vi "Save_Universal.vi"(9 "Directory Path":path=path "I:/Temporary", 11 "Data to be Save":variant[](array[variant])=[variant(string "")]) -> ()   [LabVIEW 2020]
uses:
  <vilib>/Utility/Data Type/Type Definitions/Data Type.ctl
  <vilib>/Utility/file.llb/Write Delimited Spreadsheet (DBL).vi
  <vilib>/Utility/file.llb/Write Delimited Spreadsheet (I64).vi
  <vilib>/Utility/Data Type/NI_Data Type.lvlib
panel:
  out "Array 2":T1[](array[typedef])
  out "name":string="Stringde"
  out "error out":errorcluster={"status"=TRUE, "code"=7, "source"="Open/Create/Replace File in Save_Universal.vi<APPEND>\n2021_09_06 17_44_50.md:\\"}
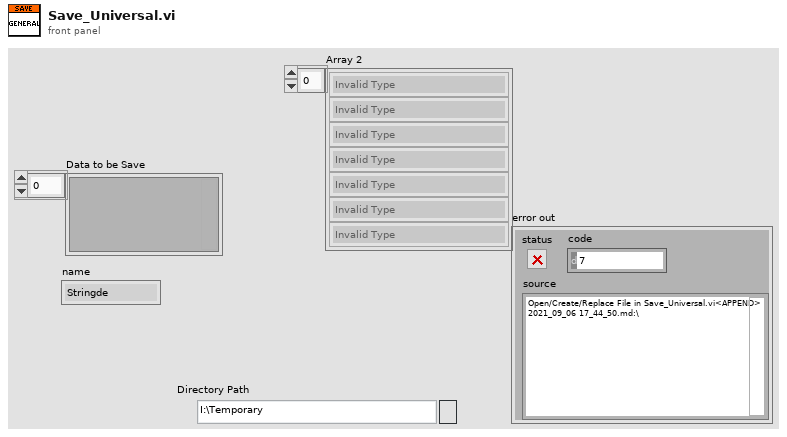
[diagram p1: front panel]
types:
  T1 = typedef "NI_Data Type.lvlib/Data Type.ctl" = enum8{"Invalid Type", "Void", "I8", "I16", "I32", "I64", "U8", "U16", "U32", "U64", "Single Float", "Double Float", "Extended Float", "Single Complex", "Double Complex", "Extended Complex", "Enum U8", "Enum U16", "Enum U32", "Enum U64", "Single Float With Unit", "Double Float With Unit", "Extended Float With Unit", "Single Complex with Unit", "Double Complex with Unit", "Extended Complex with Unit", "Boolean", "String", "Path", "Picture", "Tag", "Array", "Cluster", "Variant", "LV Variant", "Waveform", "Timestamp", "Digital Waveform", "Digital Data", "ExpressData", "Refnum", "External Data", "VI", "Poly VI", "LabVIEW Class Instance", "Fixed Point", "Set Collection", "Map Collection"}
  T2 = enum16{"open", "replace", "create", "open or create", "replace or create", "replace or create with confirmation"}
  T3 = typedef "NI_Data Type.lvlib/Refnum Type.ctl" = enum16{"NotARefnum", "UnknownRefnum", "Generic", "Datalog", "ByteStream", "Device", "Occurence", "TCPNetConnection", "Auto", "Menu", "Imaq", "Hardware", "DataSocket", "Visa", "IVI", "UDPNetConnection", "Notifier", "Queue", "Irda", "EventReg", "DotNet", "UserEvent", "Callback", "UNUSED_EMPTY_POSITION", "BlueToothNetConnection", "LVObjApp", "LVObjVI", "LVObjUnknown", "GenericClass", "UserDefinedRefnumTag", "DataValue", "RT FIFO", "TDMS File", "PythonSessionRefnum"}
  T4 = typedef "imagedata.ctl" = cluster{"image type":i32, "image depth":i32, "image":u8[], "mask":u8[], "colors":u32[], "Rectangle":cluster{"left":i16, "top":i16, "right":i16, "bottom":i16}}
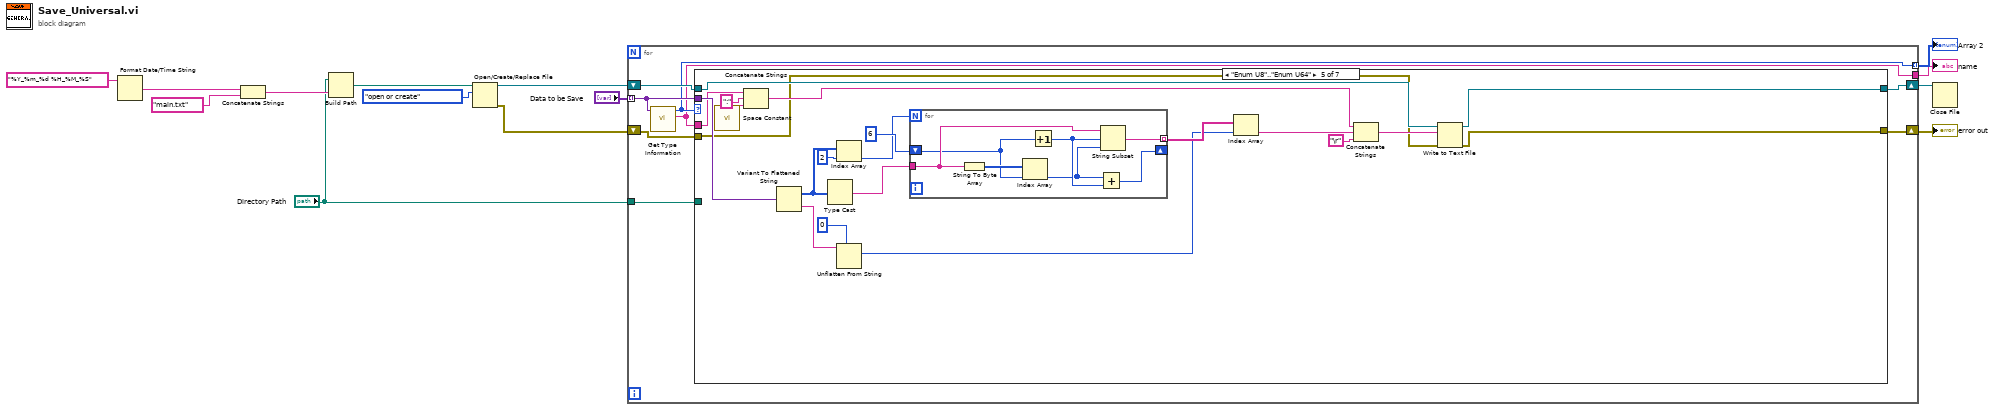
[diagram p0: block diagram]
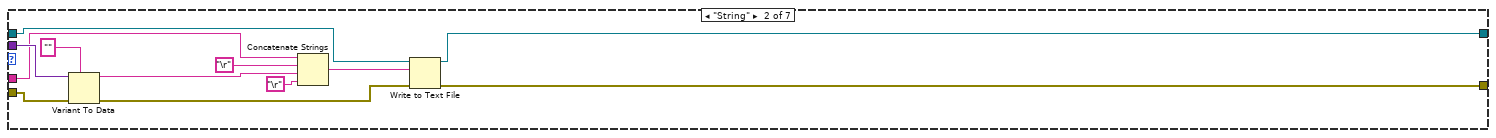
[diagram p3: hidden frame]
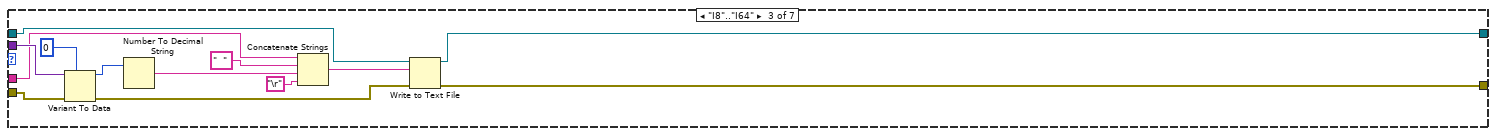
[diagram p4: hidden frame]
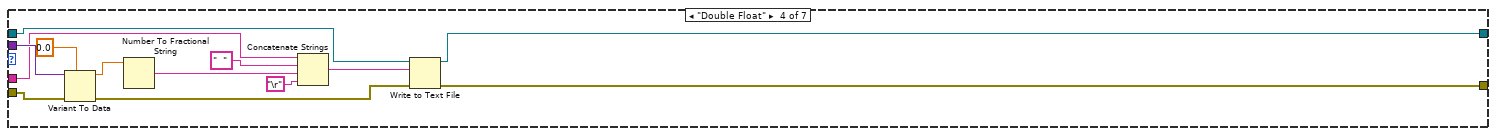
[diagram p5: hidden frame]
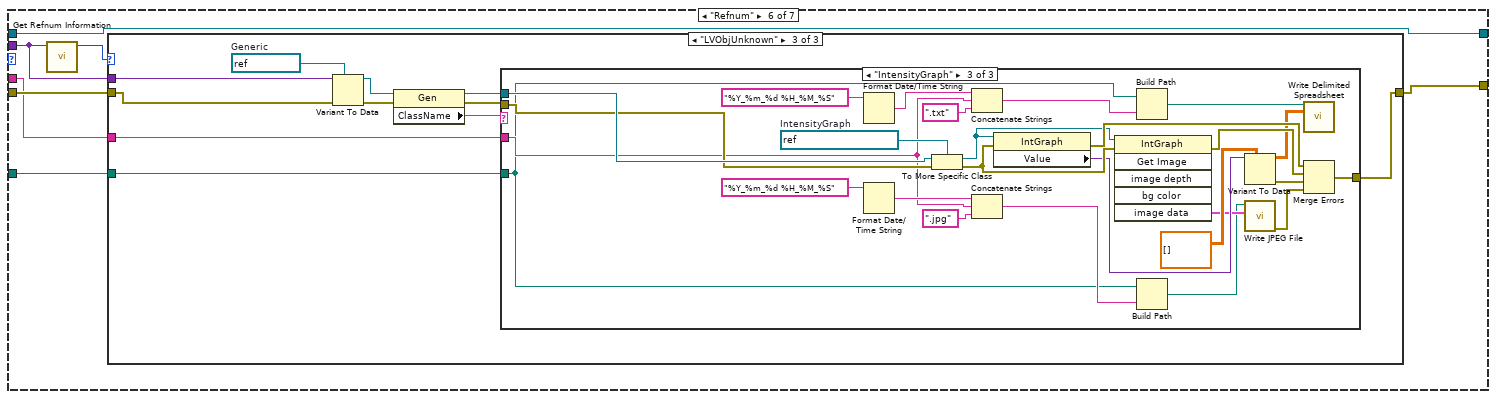
[diagram p6: hidden frame]
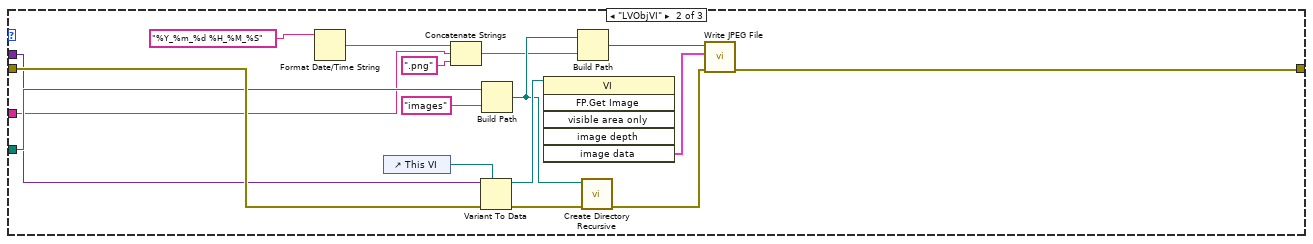
[diagram p8: hidden frame]
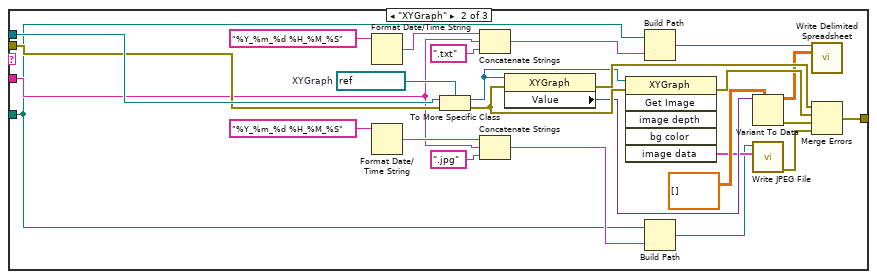
[diagram p10: hidden frame]
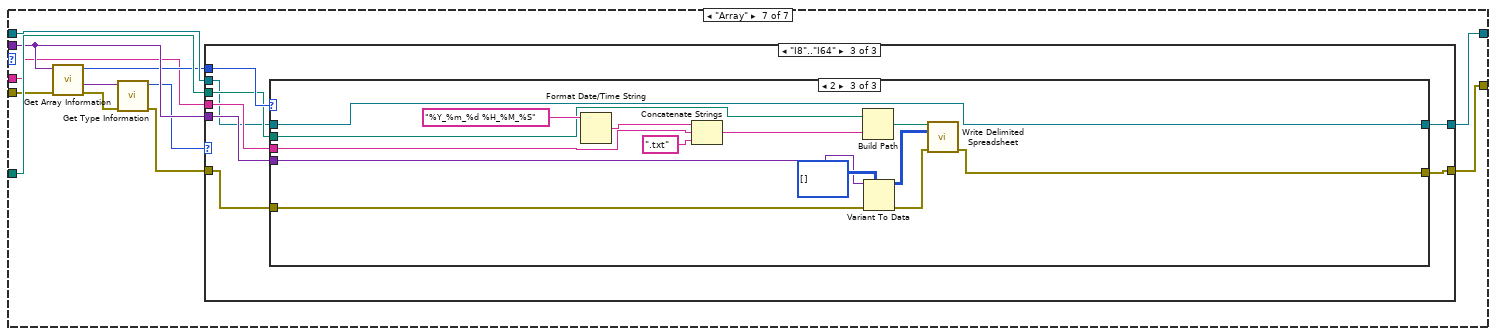
[diagram p11: hidden frame]
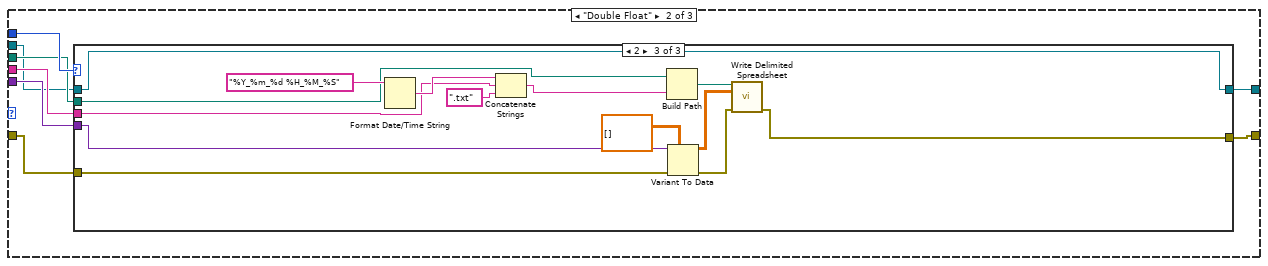
[diagram p13: hidden frame]
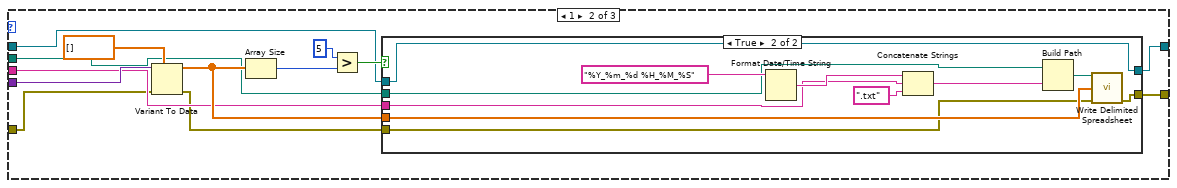
[diagram p15: hidden frame]
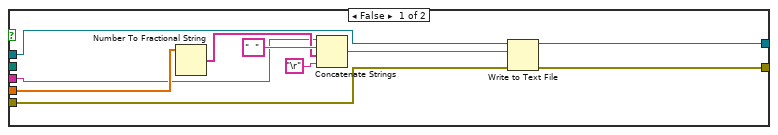
[diagram p16: hidden frame]
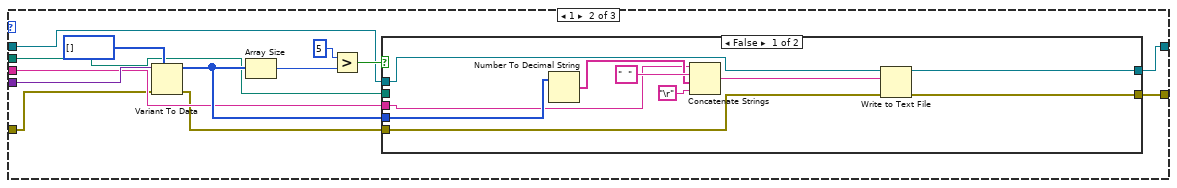
[diagram p18: hidden frame]
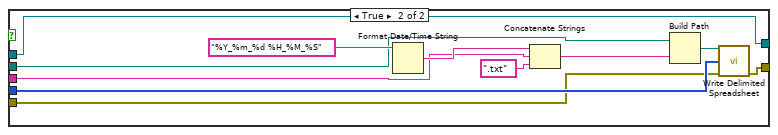
[diagram p19: hidden frame]
diagram:
  n1 = Format Date/Time String(time format string (%c)="%Y_%m_%d %H_%M_%S") -> (date/time string=w11:string)  [unwired: 2 in]
  n2 = Concatenate Strings(w11, "main.txt" ("string")) -> (w9:string)
  n3 = Build Path(base path="Directory Path", name or relative path=w9) -> (appended path=w10:path)
  n4 = Open/Create/Replace File(file path (use dialog)=w10, operation (0:open)=T2."open or create") -> (refnum out=w8:refnum<file>, error out=w7:errorcluster)  [unwired: 4 in, 1 out]
  n5 = for {
    tunnel: "Data to be Save" -> [w21] mode=indexing
    shift-right: [w19] -> w4
    shift-left: w8 -> [w22]
    shift-right: [w18] -> w6
    shift-left: w7 -> [w20]
    tunnel: "Directory Path" -> [w17]
    tunnel: [w16] -> w2 mode=indexing
    tunnel: [w15] -> w1
    n6 = call <vilib>:"Get Type Information.vi"("variant"=w21) -> ("name"=w15:string, "type"=w16:T1)  [unwired: 6 in, 3 out]
    n7 = case shown="\"Enum U8\"..\"Enum U64\"" w16 {
      tunnel: w15 -> [_ w33 w39 w54 w65 w91 w181]
      tunnel: w22 -> [w24 w30 w43 w58 w83 w94 w184]
      tunnel: w21 -> [_ w35 w47 w60 w68 w92 w188]
      tunnel: w20 -> [w23 w34 w42 w57 w63 w97 w180]
      tunnel: [w24 w28 w40 w55 w82 w94 w183] -> w19
      tunnel: [w23 w26 w41 w56 w80 w95 w189] -> w18
      tunnel: w17 -> [_ _ _ _ _ w96 w190]
      frame "Invalid Type", Default {
      }
      frame "String" {
        n8 = Variant To Data(error in=w34, type="", Variant=w35) -> (data=w32:string, error out=w27:errorcluster)
        n9 = Concatenate Strings(w33, "\r", w32, "\r") -> (w29:string)
        n10 = Write to Text File(file (use dialog)=w30, text=w29, error in=w27) -> (refnum out=w28:refnum<file>, error out=w26:errorcluster)  [unwired: 1 in, 1 out]
      }
      frame "I8".."I64" {
        n11 = Variant To Data(error in=w42, type=0, Variant=w47) -> (data=w44:i32, error out=w49:errorcluster)
        n12 = Number To Decimal String(number=w44) -> (decimal integer string=w45:string)  [unwired: 1 in]
        n13 = Concatenate Strings(w39, "  " ("string"), w45, "\r") -> (w48:string)
        n14 = Write to Text File(file (use dialog)=w43, text=w48, error in=w49) -> (refnum out=w40:refnum<file>, error out=w41:errorcluster)  [unwired: 1 in, 1 out]
      }
      frame "Double Float" {
        n15 = Variant To Data(error in=w57, type=0.0, Variant=w60) -> (data=w52:dbl, error out=w62:errorcluster)
        n16 = Number To Fractional String(number=w52) -> (F-format string=w51:string)  [unwired: 3 in]
        n17 = Concatenate Strings(w54, "  " ("string"), w51, "\r") -> (w61:string)
        n18 = Write to Text File(file (use dialog)=w58, text=w61, error in=w62) -> (refnum out=w55:refnum<file>, error out=w56:errorcluster)  [unwired: 1 in, 1 out]
      }
      frame "Enum U8".."Enum U64" {
        n19 = call <vilib>:"Space Constant.vi"() -> ("String"=w81:string)
        n20 = Concatenate Strings(w65, ":" ("string"), w81) -> (w66:string)
        n21 = Variant To Flattened String(Variant=w68) -> (data string=w77:string, 1:w71:i16[])
        n22 = Type Cast(x=w71) -> (*(type *) &x=w75:string)  [unwired: 1 in]
        n23 = Index Array(array=w71, index=2) -> (element=w69:i16)
        n24 = Unflatten From String(type=u16 0, binary string=w77) -> (value=w72:u16)  [unwired: 3 in, 2 out]
        n25 = for {
          N: w69 -> [_]
          tunnel: w75 -> [w87]
          shift-right: [w86] -> _
          shift-left: 6 ("index") -> [w84]
          tunnel: [w85] -> w73 mode=indexing
          n26 = String To Byte Array(string=w87) -> (unsigned byte array=w90:u8[])
          n27 = Index Array(array=w90, index=w84) -> (element=w88:u8)
          n28 = Increment(x=w84) -> (x+1=w89:i32)
          n29 = Add(x=w88, y=w89) -> (x+y=w86:i32)
          n30 = String Subset(string=w87, offset (0)=w89, length (rest)=w88) -> (substring=w85:string)
        }
        n31 = Index Array(array=w73, index=w72) -> (element=w67:string)
        n32 = Concatenate Strings(w66, w67, "\r") -> (w79:string)
        n33 = Write to Text File(file (use dialog)=w83, text=w79, error in=w63) -> (refnum out=w82:refnum<file>, error out=w80:errorcluster)  [unwired: 1 in, 1 out]
      }
      frame "Refnum" {
        n34 = call <vilib>:"Get Refnum Information.vi"("variant"=w92) -> ("reference type"=w93:T3)  [unwired: 7 in, 3 out]
        n35 = case shown="\"LVObjUnknown\"" w93 {
          tunnel: w97 -> [w98 w113 w123]
          tunnel: w96 -> [_ w109 w116]
          tunnel: [w98 w108 w118] -> w95
          tunnel: w92 -> [_ w107 w125]
          tunnel: w91 -> [_ w99 w117]
          frame "NotARefnum", Default {
          }
          frame "LVObjVI" {
            n36 = Format Date/Time String(time format string (%c)="%Y_%m_%d %H_%M_%S") -> (date/time string=w100:string)  [unwired: 2 in]
            n37 = control-ref of="This VI"() -> (w115:refnum<vi>)
            n38 = Concatenate Strings(w100, w99, ".png" ("string")) -> (w102:string)
            n39 = Variant To Data(error in=w113, type=w115, Variant=w107) -> (data=w112:refnum<vi>, error out=w106:errorcluster)
            n40 = Build Path(base path=w109, name or relative path="images" ("string")) -> (appended path=w104:path)
            n41 = invoke class="VI" method="FP.Get Image"(reference=w112) -> ("image data"=w114:T4)  [unwired: 5 in, 5 out]
            n42 = Build Path(base path=w104, name or relative path=w102) -> (appended path=w101:path)
            n43 = call <vilib>:"Create Directory Recursive.vi"("error in (no error)"=w106, "directory"=w104) -> ("error out"=w105:errorcluster)  [unwired: 3 in, 2 out]
            n44 = call <vilib>:"Write JPEG File.vi"("error in (no error)"=w105, "image data"=w114, "path to JPEG file"=w101) -> ("error out"=w108:errorcluster)  [unwired: 8 out]
          }
          frame "LVObjUnknown" {
            w126 = refnum<vi> refnum  # Generic
            n45 = Variant To Data(error in=w123, type=w126, Variant=w125) -> (data=w124:refnum<vi>, error out=w122:errorcluster)
            n46 = property class="Gen"(reference=w124, error in=w122) -> (reference out=w120:refnum<vi>, error out=w119:errorcluster, "ClassName"=w121:string)
            n47 = case shown="\"IntensityGraph\"" w121 {
              tunnel: w120 -> [_ w151 w177]
              tunnel: w119 -> [_ w150 w176]
              tunnel: [_ w146 w172] -> w118
              tunnel: w117 -> [_ w133 w159]
              tunnel: w116 -> [_ w130 w156]
              frame "False", Default {
              }
              frame "XYGraph" {
                w152 = refnum<vi> refnum  # XYGraph
                n48 = Format Date/Time String(time format string (%c)="%Y_%m_%d %H_%M_%S") -> (date/time string=w138:string)  [unwired: 2 in]
                n49 = Format Date/Time String(time format string (%c)="%Y_%m_%d %H_%M_%S") -> (date/time string=w135:string)  [unwired: 2 in]
                n50 = To More Specific Class(target class=w152, reference=w151, error in=w150) -> (specific class reference=w145:refnum<vi>, error out=w149:errorcluster)
                n51 = Concatenate Strings(w138, w133, ".txt" ("string")) -> (w136:string)
                n52 = Concatenate Strings(w135, w133, ".jpg" ("string")) -> (w131:string)
                n53 = property class="XYGraph"(reference=w145, error in=w149) -> (error out=w148:errorcluster, "Value"=w144:variant)  [unwired: 1 out]
                n54 = invoke class="XYGraph" method="Get Image"(reference=w145, error in=w149) -> (error out=w147:errorcluster, "image data"=w132:T4)  [unwired: 4 in, 4 out]
                n55 = Build Path(base path=w130, name or relative path=w136) -> (appended path=w137:path)
                n56 = Build Path(base path=w130, name or relative path=w131) -> (appended path=w129:path)
                n57 = Variant To Data(type=dbl[][] [] ("1D data"), Variant=w144) -> (data=w142:dbl[][], error out=w143:errorcluster)  [unwired: 1 in]
                n58 = call <vilib>:"Write JPEG File.vi"("image data"=w132, "path to JPEG file"=w129) -> ("error out"=w128:errorcluster)  [unwired: 1 in, 8 out]
                n59 = call-poly <vilib>:"Write Delimited Spreadsheet.vi"("file path (dialog if empty)"=w137, "2D data"=w142) -> ()  [unwired: 12 in, 2 out]
                n60 = Merge Errors(w148, w147, w143, w128) -> (w146:errorcluster)
              }
              frame "IntensityGraph" {
                w178 = refnum<vi> refnum  # IntensityGraph
                n61 = Format Date/Time String(time format string (%c)="%Y_%m_%d %H_%M_%S") -> (date/time string=w164:string)  [unwired: 2 in]
                n62 = Format Date/Time String(time format string (%c)="%Y_%m_%d %H_%M_%S") -> (date/time string=w161:string)  [unwired: 2 in]
                n63 = To More Specific Class(target class=w178, reference=w177, error in=w176) -> (specific class reference=w171:refnum<vi>, error out=w175:errorcluster)
                n64 = Concatenate Strings(w164, w159, ".txt" ("string")) -> (w162:string)
                n65 = Concatenate Strings(w161, w159, ".jpg" ("string")) -> (w157:string)
                n66 = property class="IntGraph"(reference=w171, error in=w175) -> (error out=w174:errorcluster, "Value"=w170:variant)  [unwired: 1 out]
                n67 = invoke class="IntGraph" method="Get Image"(reference=w171, error in=w175) -> (error out=w173:errorcluster, "image data"=w158:T4)  [unwired: 4 in, 4 out]
                n68 = Build Path(base path=w156, name or relative path=w162) -> (appended path=w163:path)
                n69 = Build Path(base path=w156, name or relative path=w157) -> (appended path=w155:path)
                n70 = Variant To Data(type=dbl[][] [] ("1D data"), Variant=w170) -> (data=w168:dbl[][], error out=w169:errorcluster)  [unwired: 1 in]
                n71 = call <vilib>:"Write JPEG File.vi"("image data"=w158, "path to JPEG file"=w155) -> ("error out"=w154:errorcluster)  [unwired: 1 in, 8 out]
                n72 = call-poly <vilib>:"Write Delimited Spreadsheet.vi"("file path (dialog if empty)"=w163, "2D data"=w168) -> ()  [unwired: 12 in, 2 out]
                n73 = Merge Errors(w174, w173, w169, w154) -> (w172:errorcluster)
              }
            }
          }
        }
      }
      frame "Array" {
        n74 = call <vilib>:"Get Array Information.vi"("error in (no error)"=w180, "variant"=w188) -> ("error out"=w187:errorcluster, "array element data type"=w186:variant, "number of dimensions"=w182:i32)  [unwired: 6 in, 1 out]
        n75 = call <vilib>:"Get Type Information.vi"("error in (no error)"=w187, "variant"=w186) -> ("error out"=w179:errorcluster, "type"=w185:T1)  [unwired: 5 in, 3 out]
        n76 = case shown="\"I8\"..\"I64\"" w185 {
          tunnel: w179 -> [w192 w196 w254]
          tunnel: w190 -> [_ w198 w256]
          tunnel: [w192 w195 w253] -> w189
          tunnel: w188 -> [_ w197 w255]
          tunnel: w184 -> [w191 w193 w251]
          tunnel: [w191 w194 w252] -> w183
          tunnel: w182 -> [_ w200 w258]
          tunnel: w181 -> [_ w199 w257]
          frame "Invalid Type", Default {
          }
          frame "Double Float" {
            n77 = case shown="2" w200 {
              tunnel: w199 -> [_ w208 w248]
              tunnel: w198 -> [_ w209 w245]
              tunnel: w197 -> [_ w214 w242]
              tunnel: w196 -> [w201 w206 w241]
              tunnel: [w201 w204 w238] -> w195
              tunnel: w193 -> [w202 w207 w237]
              tunnel: [w202 w203 w237] -> w194
              frame 0, Default {
              }
              frame 1 {
                n78 = Variant To Data(error in=w206, type=dbl[] [] ("1D data"), Variant=w214) -> (data=w210:dbl[], error out=w205:errorcluster)
                n79 = Array Size(array=w210) -> (size(s)=w213:i32)
                n80 = Greater?(x=5, y=w213) -> (0:w211:bool)
                n81 = case shown="True" w211 {
                  tunnel: w210 -> [w221 w236]
                  tunnel: w209 -> [_ w231]
                  tunnel: w208 -> [w218 w229]
                  tunnel: w207 -> [w217 w228]
                  tunnel: w205 -> [w220 w227]
                  tunnel: [w219 w226] -> w204
                  tunnel: [w216 w228] -> w203
                  frame False {
                    n82 = Number To Fractional String(number=w221) -> (F-format string=w223:string[])  [unwired: 3 in]
                    n83 = Concatenate Strings(w218, "  " ("string"), w223, "\r") -> (w225:string)
                    n84 = Write to Text File(file (use dialog)=w217, text=w225, error in=w220) -> (refnum out=w216:refnum<file>, error out=w219:errorcluster)  [unwired: 1 in, 1 out]
                  }
                  frame True {
                    n85 = Format Date/Time String(time format string (%c)="%Y_%m_%d %H_%M_%S") -> (date/time string=w235:string)  [unwired: 2 in]
                    n86 = Concatenate Strings(w235, w229, ".txt" ("string")) -> (w232:string)
                    n87 = Build Path(base path=w231, name or relative path=w232) -> (appended path=w230:path)
                    n88 = call-poly <vilib>:"Write Delimited Spreadsheet.vi"("file path (dialog if empty)"=w230, "1D data"=w236, "error in (no error)"=w227) -> ("error out"=w226:errorcluster)  [unwired: 11 in, 1 out]
                  }
                }
              }
              frame 2 {
                n89 = Format Date/Time String(time format string (%c)="%Y_%m_%d %H_%M_%S") -> (date/time string=w250:string)  [unwired: 2 in]
                n90 = Concatenate Strings(w250, w248, ".txt" ("string")) -> (w244:string)
                n91 = Build Path(base path=w245, name or relative path=w244) -> (appended path=w246:path)
                n92 = Variant To Data(error in=w241, type=dbl[][] [] ("2D data"), Variant=w242) -> (data=w239:dbl[][], error out=w240:errorcluster)
                n93 = call-poly <vilib>:"Write Delimited Spreadsheet.vi"("file path (dialog if empty)"=w246, "2D data"=w239, "error in (no error)"=w240) -> ("error out"=w238:errorcluster)  [unwired: 11 in, 1 out]
              }
            }
          }
          frame "I8".."I64" {
            n94 = case shown="2" w258 {
              tunnel: w257 -> [_ w266 w306]
              tunnel: w256 -> [_ w267 w303]
              tunnel: w255 -> [_ w272 w300]
              tunnel: w254 -> [w259 w264 w299]
              tunnel: [w259 w262 w296] -> w253
              tunnel: w251 -> [w260 w265 w295]
              tunnel: [w260 w261 w295] -> w252
              frame 0, Default {
              }
              frame 1 {
                n95 = Variant To Data(error in=w264, type=i32[] [] ("1D data"), Variant=w272) -> (data=w268:i32[], error out=w263:errorcluster)
                n96 = Array Size(array=w268) -> (size(s)=w271:i32)
                n97 = Greater?(x=5, y=w271) -> (0:w269:bool)
                n98 = case shown="False" w269 {
                  tunnel: w268 -> [w279 w294]
                  tunnel: w267 -> [_ w289]
                  tunnel: w266 -> [w276 w287]
                  tunnel: w265 -> [w275 w286]
                  tunnel: w263 -> [w278 w285]
                  tunnel: [w277 w284] -> w262
                  tunnel: [w274 w286] -> w261
                  frame False {
                    n99 = Number To Decimal String(number=w279) -> (decimal integer string=w281:string[])  [unwired: 1 in]
                    n100 = Concatenate Strings(w276, "  " ("string"), w281, "\r") -> (w283:string)
                    n101 = Write to Text File(file (use dialog)=w275, text=w283, error in=w278) -> (refnum out=w274:refnum<file>, error out=w277:errorcluster)  [unwired: 1 in, 1 out]
                  }
                  frame True {
                    n102 = Format Date/Time String(time format string (%c)="%Y_%m_%d %H_%M_%S") -> (date/time string=w293:string)  [unwired: 2 in]
                    n103 = Concatenate Strings(w293, w287, ".txt" ("string")) -> (w290:string)
                    n104 = Build Path(base path=w289, name or relative path=w290) -> (appended path=w288:path)
                    n105 = call-poly <vilib>:"Write Delimited Spreadsheet.vi"("file path (dialog if empty)"=w288, "1D data"=w294, "error in (no error)"=w285) -> ("error out"=w284:errorcluster)  [unwired: 11 in, 1 out]
                  }
                }
              }
              frame 2 {
                n106 = Format Date/Time String(time format string (%c)="%Y_%m_%d %H_%M_%S") -> (date/time string=w308:string)  [unwired: 2 in]
                n107 = Concatenate Strings(w308, w306, ".txt" ("string")) -> (w302:string)
                n108 = Build Path(base path=w303, name or relative path=w302) -> (appended path=w304:path)
                n109 = Variant To Data(error in=w299, type=i32[][] [] ("2D data"), Variant=w300) -> (data=w297:i32[][], error out=w298:errorcluster)
                n110 = call-poly <vilib>:"Write Delimited Spreadsheet.vi"("file path (dialog if empty)"=w304, "2D data"=w297, "error in (no error)"=w298) -> ("error out"=w296:errorcluster)  [unwired: 11 in, 1 out]
              }
            }
          }
        }
      }
    }
  }
  "error out" <- w6
  "Array 2" <- w2
  "name" <- w1
  n111 = Close File(refnum=w4) -> ()  [unwired: 1 in, 2 out]
